vi "PWM FPGA.vi"(7 "引用句柄输入":refnum<k21>, 10 "F":u32, 11 "T":u32) -> ()   [LabVIEW 2017]
uses:
  <vilib>/rvi/eio/common/nirviEmuTemplateMethod_errors.vi
  <vilib>/eio/EIONode/EIONode.xnode
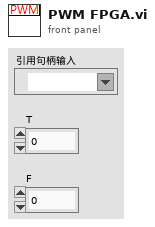
[diagram p1: front panel]
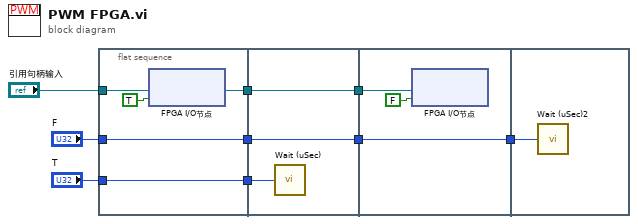
[diagram p0: block diagram]
diagram:
  n1 = flat-sequence {
    tunnel: "引用句柄输入" -> [w14]
    tunnel: [w13] -> w9
    tunnel: "T" -> [w12]
    tunnel: [w12] -> w8
    tunnel: "F" -> [w11]
    tunnel: [w11] -> w7
    tunnel: w9 -> [w17]
    tunnel: w8 -> [w16]
    tunnel: [w17] -> w6
    tunnel: w7 -> [w15]
    tunnel: [w15] -> w5
    tunnel: w6 -> [w20]
    tunnel: w5 -> [w19]
    tunnel: [w19] -> w4
    tunnel: w4 -> [w21]
    frame #0 {
      n2 = xnode "FPGA I/O节点"("I/O项"=TRUE ("invert pulse (F)"), "FPGA I/O输入"=w14) -> ("FPGA I/O输出"=w13:refnum<k21>)
    }
    frame #1 {
      n3 = call "Wait (uSec)"("Count(uSec)"=w16) -> ()  [unwired: 1 out]
    }
    frame #2 {
      n4 = xnode "FPGA I/O节点"("I/O项"=FALSE ("invert pulse (F)"), "FPGA I/O输入"=w20) -> ()  [unwired: 1 out]
    }
    frame #3 {
      n5 = call "Wait (uSec)2"("Count(uSec)"=w21) -> ()  [unwired: 1 out]
    }
  }
